vi "sub_heading_line_simul.vi"(8 "error in":errorcluster, 11 "Heading":dbl) -> (0 "error out":errorcluster, 3 "heading_curr":cluster{dbl, dbl}[](array[cluster]))   [LabVIEW 2019]
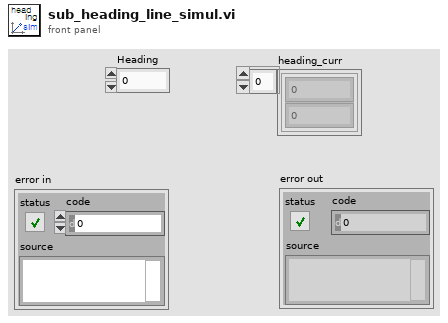
[diagram p1: front panel]
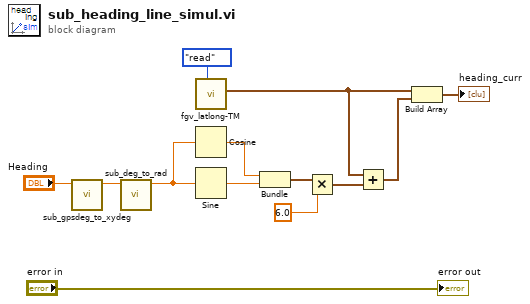
[diagram p0: block diagram]
diagram:
  n1 = call "sub_gpsdeg_to_xydeg.vi"("Heading"="Heading") -> ("deg"=w8:dbl)  [unwired: 10 in]
  n2 = call "sub_deg_to_rad.vi"("deg in"=w8) -> ("rad out"=w9:dbl)  [unwired: 10 in]
  n3 = call "fgv_latlong-TM.vi"("cmd"=enum16{"write", "read"}."read") -> ("latlong out"=w1:cluster{dbl, dbl})  [unwired: 9 in, 1 out]
  n4 = Cosine(x=w9) -> (cos(x)=w10:dbl)
  n5 = Sine(x=w9) -> (sin(x)=w11:dbl)
  n6 = Bundle(w10, w11) -> (w4:cluster{dbl, dbl})  [unwired: 1 in]
  n7 = Multiply(x=w4, y=6.0) -> (x*y=w3:cluster{dbl, dbl})
  n8 = Add(x=w1, y=w3) -> (x+y=w13:cluster{dbl, dbl})
  n9 = Build Array(w1, w13) -> (→"heading_curr":cluster{dbl, dbl}[])
  "error out" <- "error in"
